vi "Fire_BurstPuls_nowait.vi"(1 "error in":errorcluster, 2 "milliseconds to wait":u32) -> (0 "error out":errorcluster)   [LabVIEW 2016]
uses:
  Utility/Global_Laser.vi
  Program Files (x86)/OPOTEK_DLL/OPOTEK.dll
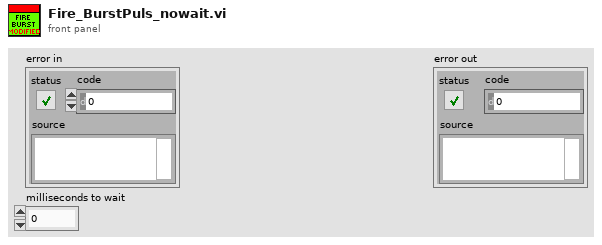
[diagram p1: front panel]
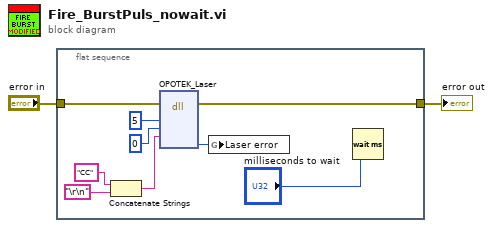
[diagram p0: block diagram]
diagram:
  n1 = flat-sequence {
    tunnel: [w11] -> w1
    tunnel: "error in" -> [w4]
    frame #0 {
      n2 = Concatenate Strings("CC", "\r\n") -> (w10:string)
      n3 = dll-call lib="C:/Program Files (x86)/OPOTEK_DLL/OPOTEK.dll" fn="OPOTEK_Laser"(error in=w4, "action"=i8 5, "parameter"=i16 0, "stringToSend"=w10) -> (error out=w11:errorcluster, "error_Code"=w6:i32)  [unwired: 7 in, 1 out]
      n4 = global write "Global_Laser.vi" "Laser error"(w6) -> ()
      n5 = Wait (ms)(milliseconds to wait="milliseconds to wait") -> ()  [unwired: 1 out]
    }
  }
  "error out" <- w1
